vi "Dynamic Data Builder.vi"(9 "Signal Name":string, 10 "Unit":string, 11 "Number in":dbl) -> (2 "Dynamic Signame Out":dynamicdata(graph))   [LabVIEW 2014, in "Data Saving.lvlib" / "Data Saver.lvclass"]
uses:
  Data Saver.lvclass
  <vilib>/express/express signal manip/GetorSetDDTAttributes/Shared VIs/TimeType.ctl
  <vilib>/express/express signal manip/GetorSetDDTAttributes/Shared VIs/XDimension.ctl
  <vilib>/express/express signal manip/GetorSetDDTAttributes/Shared VIs/TimeMode Enum to Boolean.vi
  <vilib>/express/express signal manip/GetorSetDDTAttributes/Shared VIs/XDimension Enum to String.vi
  <vilib>/express/express shared/transition.llb/Dynamic To Waveform Array.vi
  <vilib>/express/express signal manip/GetorSetDDTAttributes/Set DDT Attributes/SetT0.vi
  <vilib>/express/express shared/transition.llb/Waveform Array To Dynamic.vi
  <vilib>/express/express signal manip/GetorSetDDTAttributes/Set DDT Attributes/Set DDT Properties.xnode
  <vilib>/express/express signal manip/GetorSetDDTAttributes/Shared VIs/GetSetShared.lvlib
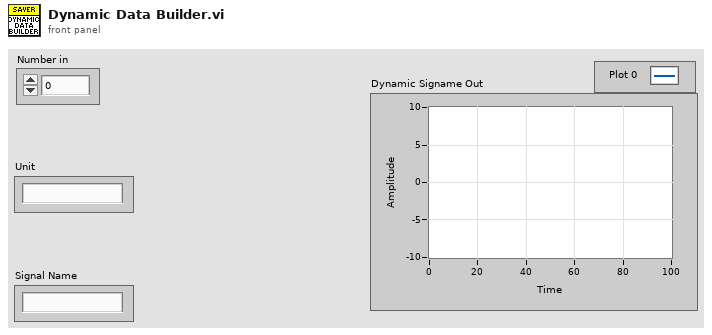
[diagram p1: front panel]
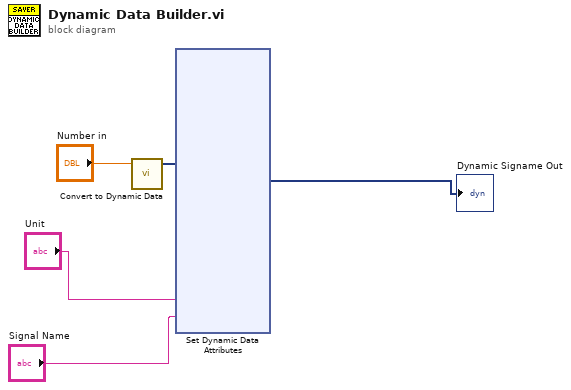
[diagram p0: block diagram]
diagram:
  n1 = call "Convert to Dynamic Data"("Double"="Number in") -> ("Dynamic Data Type"=w4:dynamicdata)  [unwired: 3 in]
  n2 = xnode "Set Dynamic Data Attributes"("Signals In"=w4, "Unit"="Unit", "Signal Name"="Signal Name") -> ("Signals Out"=→"Dynamic Signame Out":dynamicdata)  [unwired: 5 in, 1 out]
